vi "xml.scalar.vi"(10 "Value":variant, 11 "MsgSerializer.XML in":refnum<class "MsgSerializer.XML.lvclass">) -> (2 "error out":errorcluster, 3 "string":string)   [LabVIEW 2013, in "Caraya.lvlib" / "MsgSerializer.XML.lvclass"]
uses:
  MsgSerializer.XML.lvclass
  MsgSerializer/MsgSerializer.lvclass/MsgSerializer.ctl
  MsgSerializer.XML.lvclass/MsgSerializer.XML.ctl
  MsgSerializer/MsgSerializer.lvclass
  <vilib>/Utility/VariantDataType/VariantType.lvlib
  Caraya.lvlib
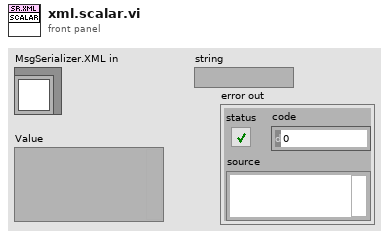
[diagram p1: front panel]
types:
  T1 = typedef "VariantType.lvlib/Type.ctl" = enum8{"Invalid Type", "Void", "I8", "I16", "I32", "I64", "U8", "U16", "U32", "U64", "Single Float", "Double Float", "Extended Float", "Single Complex", "Double Complex", "Extended Complex", "Enum U8", "Enum U16", "Enum U32", "Enum U64", "Single Float With Unit", "Double Float With Unit", "Extended Float With Unit", "Single Complex with Unit", "Double Complex with Unit", "Extended Complex with Unit", "Boolean", "String", "Path", "Picture", "Tag", "Array", "Cluster", "Variant", "LV Variant", "Waveform", "Timestamp", "Digital Waveform", "Digital Data", "ExpressData", "Refnum", "External Data", "VI", "Poly VI", "LabVIEW Class Instance", "Fixed Point"}
  T2 = typedef "Caraya.lvlib/MsgSerializer.lvclass/decimal-notation -- enum.ctl" = enum16{"System-defined", "dot-notation", "comma-notation"}
  T3 = typedef "Caraya.lvlib/MsgSerializer.XML.lvclass/format -- enum.ctl" = enum16{"value", "tag", "property"}
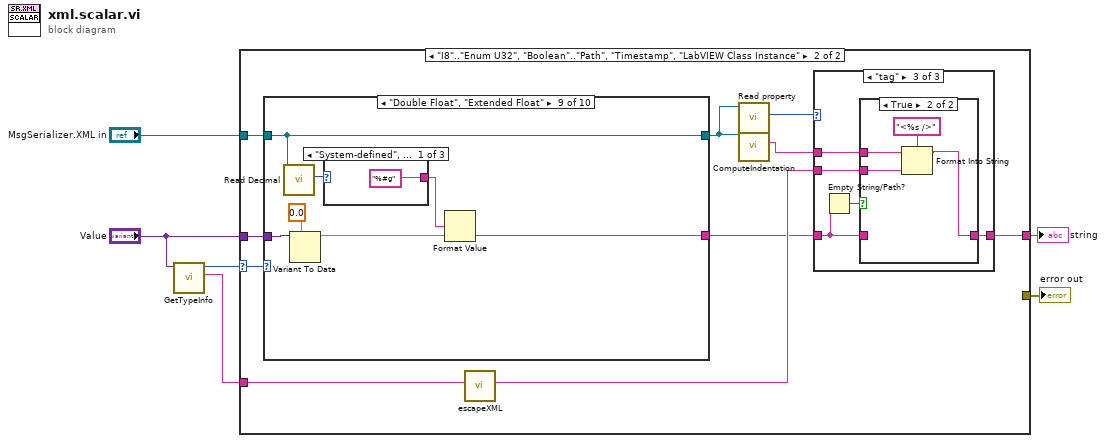
[diagram p0: block diagram]
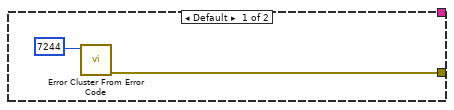
[diagram p2: hidden frame]
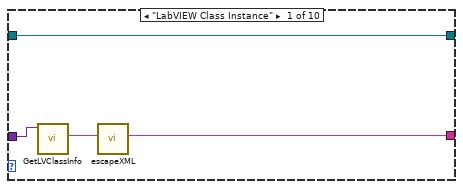
[diagram p3: hidden frame]
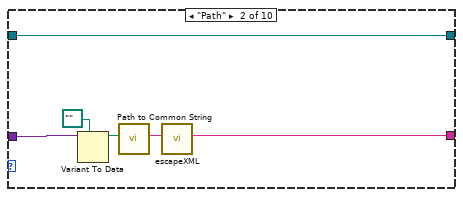
[diagram p4: hidden frame]
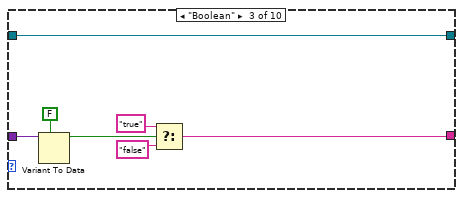
[diagram p5: hidden frame]
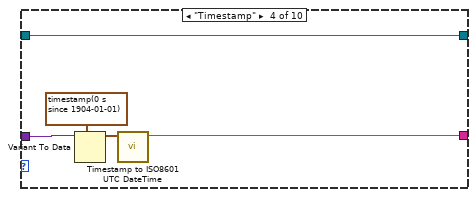
[diagram p6: hidden frame]
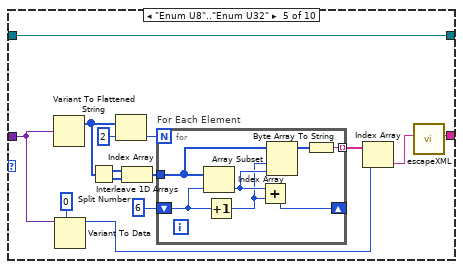
[diagram p7: hidden frame]
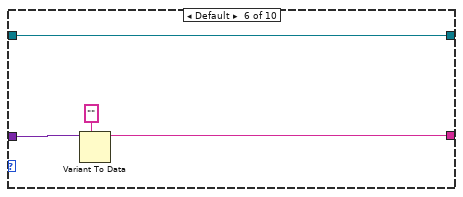
[diagram p8: hidden frame]
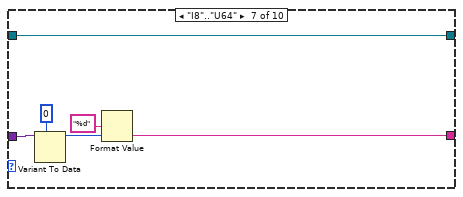
[diagram p9: hidden frame]
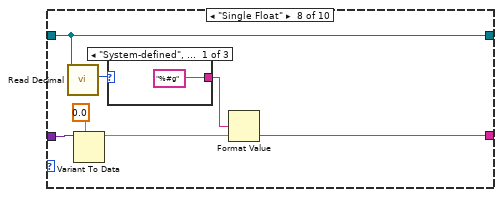
[diagram p10: hidden frame]
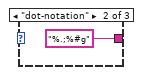
[diagram p11: hidden frame]
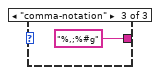
[diagram p12: hidden frame]
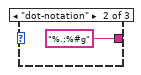
[diagram p13: hidden frame]
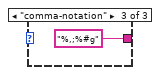
[diagram p14: hidden frame]
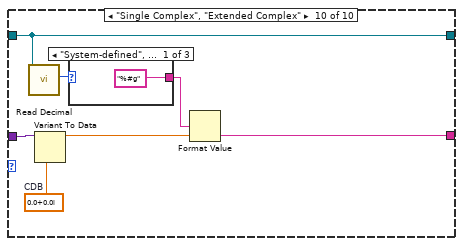
[diagram p15: hidden frame]
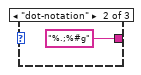
[diagram p16: hidden frame]
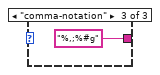
[diagram p17: hidden frame]
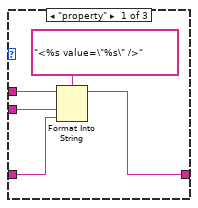
[diagram p18: hidden frame]
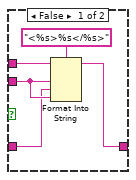
[diagram p20: hidden frame]
diagram:
  n1 = call <vilib>:"GetTypeInfo.vi"("Variant"="Value") -> ("Name"=w5:string, "Type Enum"=w2:T1)  [unwired: 6 in, 3 out]
  n2 = case shown="\"I8\"..\"Enum U32\", \"Boolean\"..\"Path\", \"Timestamp\", \"LabVIEW Class Instance\"" w2 {
    selector: w2 -> [_ w12]
    tunnel: "Value" -> [_ w13]
    tunnel: w5 -> [_ w16]
    tunnel: "MsgSerializer.XML in" -> [_ w10]
    tunnel: [_ w14] -> w3
    tunnel: [w7 _] -> w1
    frame Default {
      n3 = call <vilib>:"Error Cluster From Error Code.vi"("error code (0)"=7244) -> ("error out"=w7:errorcluster)  [unwired: 8 in]
    }
    frame "I8".."Enum U32", "Boolean".."Path", "Timestamp", "LabVIEW Class Instance" {
      n4 = case shown="\"Double Float\", \"Extended Float\"" w12 {
        tunnel: w13 -> [w22 w26 w30 w37 w44 w64 w68 w77 w87 w97]
        tunnel: [w20 w24 w29 w38 w42 w63 w67 w76 w86 w96] -> w11
        tunnel: w10 -> [w19 w23 w35 w36 w41 w62 w66 w74 w84 w95]
        tunnel: [w19 w23 w35 w36 w41 w62 w66 w74 w84 w95] -> w9
        frame "LabVIEW Class Instance" {
          n5 = call <vilib>:"GetLVClassInfo.vi"("Variant"=w22) -> ("LV Class File Name"=w21:string)  [unwired: 8 in, 2 out]
          n6 = call "escapeXML.vi"("Input String"=w21) -> ("XML-escaped String"=w20:string)  [unwired: 10 in]
        }
        frame "Path" {
          n7 = Variant To Data(type=path "", Variant=w26) -> (data=w27:path)  [unwired: 1 in, 1 out]
          n8 = call "Path to Common String.vi"("specific path"=w27) -> ("common path"=w25:string)  [unwired: 10 in]
          n9 = call "escapeXML.vi"("Input String"=w25) -> ("XML-escaped String"=w24:string)  [unwired: 10 in]
        }
        frame "Boolean" {
          n10 = Variant To Data(type=FALSE, Variant=w30) -> (data=w31:bool)  [unwired: 1 in, 1 out]
          n11 = Select(t="true", s=w31, f="false") -> (s? t:f=w29:string)
        }
        frame "Timestamp" {
          n12 = Variant To Data(type=timestamp(0 s since 1904-01-01) ("current time"), Variant=w37) -> (data=w39:timestamp)  [unwired: 1 in, 1 out]
          n13 = call <vilib>:"Timestamp to ISO8601 UTC DateTime.vi"("Timestamp (now)"=w39) -> ("ISO8601 UTC DateTime"=w38:string)  [unwired: 10 in]
        }
        frame "Enum U8".."Enum U32" {
          n14 = Variant To Flattened String(Variant=w44) -> (1:w46:i16[])  [unwired: 1 out]
          n15 = Variant To Data(type=u32 0, Variant=w44) -> (data=w45:u32)  [unwired: 1 in, 1 out]
          n16 = Split Number(x=w46) -> (hi(x)=w51:u8[], lo(x)=w50:u8[])
          n17 = Index Array(array=w46, index=2) -> (element=w53:i16)
          n18 = Interleave 1D Arrays(w51, w50) -> (w49:u8[])
          n19 = for "For Each Element" {
            N: w53 -> [_]
            shift-right: [w58] -> _
            shift-left: 6 ("index") -> [w61]
            tunnel: w49 -> [w59]
            tunnel: [w56] -> w47 mode=indexing
            n20 = Index Array(array=w59, index=w61) -> (element=w57:u8)
            n21 = Increment(x=w61) -> (x+1=w55:i32)
            n22 = Add(x=w57, y=w55) -> (x+y=w58:i32)
            n23 = Array Subset(array=w59, index=w55, length=w57) -> (w60:u8[])
            n24 = Byte Array To String(unsigned byte array=w60) -> (string=w56:string)
          }
          n25 = Index Array(array=w47, index=w45) -> (element=w43:string)
          n26 = call "escapeXML.vi"("Input String"=w43) -> ("XML-escaped String"=w42:string)  [unwired: 10 in]
        }
        frame Default {
          n27 = Variant To Data(type="", Variant=w64) -> (data=w63:string)  [unwired: 1 in, 1 out]
        }
        frame "I8".."U64" {
          n28 = Variant To Data(type=i64 0, Variant=w68) -> (data=w69:i64)  [unwired: 1 in, 1 out]
          n29 = Format Value(format string="%d", value (0)=w69) -> (output string=w67:string)  [unwired: 1 in]
        }
        frame "Single Float" {
          n30 = call "Read Decimal.vi"("MsgSerializer"=w74) -> ("Decimal"=w73:T2)  [unwired: 9 in, 1 out]
          n31 = Variant To Data(type=sgl 0.0, Variant=w77) -> (data=w78:sgl)  [unwired: 1 in, 1 out]
          n32 = case shown="\"System-defined\", Default" w73 {
            tunnel: ["%#g" ("format string") "%.;%#g" ("format string") "%,;%#g" ("format string")] -> w72
            frame "System-defined", Default {
            }
            frame "dot-notation" {
            }
            frame "comma-notation" {
            }
          }
          n33 = Format Value(format string=w72, value (0)=w78) -> (output string=w76:string)  [unwired: 1 in]
        }
        frame "Double Float", "Extended Float" {
          n34 = call "Read Decimal.vi"("MsgSerializer"=w84) -> ("Decimal"=w83:T2)  [unwired: 9 in, 1 out]
          n35 = Variant To Data(type=0.0, Variant=w87) -> (data=w88:dbl)  [unwired: 1 in, 1 out]
          n36 = case shown="\"System-defined\", Default" w83 {
            tunnel: ["%#g" ("format string") "%.;%#g" ("format string") "%,;%#g" ("format string")] -> w82
            frame "System-defined", Default {
            }
            frame "dot-notation" {
            }
            frame "comma-notation" {
            }
          }
          n37 = Format Value(format string=w82, value (0)=w88) -> (output string=w86:string)  [unwired: 1 in]
        }
        frame "Single Complex", "Extended Complex" {
          w92 = cdb 0.0+0.0i  # CDB
          n38 = call "Read Decimal.vi"("MsgSerializer"=w95) -> ("Decimal"=w94:T2)  [unwired: 9 in, 1 out]
          n39 = Variant To Data(type=w92, Variant=w97) -> (data=w98:cdb)  [unwired: 1 in, 1 out]
          n40 = case shown="\"System-defined\", Default" w94 {
            tunnel: ["%#g" ("format string") "%.;%#g" ("format string") "%,;%#g" ("format string")] -> w93
            frame "System-defined", Default {
            }
            frame "dot-notation" {
            }
            frame "comma-notation" {
            }
          }
          n41 = Format Value(format string=w93, value (0)=w98) -> (output string=w96:string)  [unwired: 1 in]
        }
      }
      n42 = call "escapeXML.vi"("Input String"=w16) -> ("XML-escaped String"=w17:string)  [unwired: 10 in]
      n43 = call "Read property.vi"("MsgSerializer.XMLProperty in"=w9) -> ("format"=w18:T3)  [unwired: 9 in, 1 out]
      n44 = call "ComputeIndentation.vi"("MsgSerializer in"=w9) -> ("indentation"=w15:string)  [unwired: 10 in]
      n45 = case shown="\"tag\"" w18 {
        tunnel: w11 -> [w105 w107 w109]
        tunnel: [w104 w107 w110] -> w14
        tunnel: w15 -> [w102 _ w112]
        tunnel: w17 -> [w103 _ w111]
        frame "property" {
          n46 = Format Into String(format string="<%s value=\"%s\" />" ("name"), initial string=w102, w103, w105) -> (resulting string=w104:string)  [unwired: 1 in, 1 out]
        }
        frame "value" {
        }
        frame "tag" {
          n47 = Empty String/Path?(string/path=w109) -> (empty?=w108:bool)
          n48 = case shown="True" w108 {
            tunnel: w112 -> [w116 w120]
            tunnel: w111 -> [w115 w118]
            tunnel: [w114 w119] -> w110
            tunnel: w109 -> [w113 _]
            frame False {
              n49 = Format Into String(format string="<%s>%s</%s>" ("name"), initial string=w116, w115, w113, w115) -> (resulting string=w114:string)  [unwired: 1 in, 1 out]
            }
            frame True {
              n50 = Format Into String(format string="<%s />" ("name"), initial string=w120, w118) -> (resulting string=w119:string)  [unwired: 1 in, 1 out]
            }
          }
        }
      }
    }
  }
  "string" <- w3
  "error out" <- w1
